vi "AppendNewPackets.vi"(6 "SampleLen":i32, 7 "SamplesInPacketNrLen":i32, 8 "ErrorIn":errorcluster, 9 "PacketsNum":u32, 10 "PacketsIn":T1[][](array[typedef]), 11 "FrameIn":string) -> (0 "ErrorOut":errorcluster, 2 "FrameOut":string, 3 "PacketsOut":T1[][](array[typedef]))   [LabVIEW 2016]
doc: "Convert input frame (string) and append new packets to the packet array. \n\nIf error occurs or is at the input, the VI ends execution."
uses:
  FallSensor/Sample.ctl
  FallSensor/Data.ctl
  FallSensor/DataType.ctl
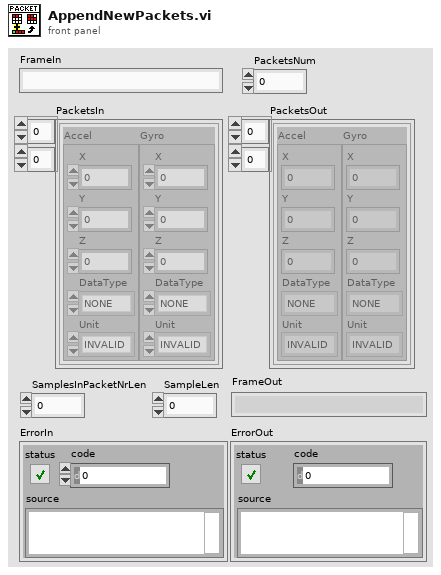
[diagram p1: front panel]
types:
  T1 = typedef "Sample.ctl" = cluster{"Accel":T2, "Gyro":T2}
  T2 = typedef "Data.ctl" = cluster{"X":dbl, "Y":dbl, "Z":dbl, "DataType":T3, "Unit":enum16{"INVALID", "g", "°/sec"}}
  T3 = typedef "DataType.ctl" = enum16{"NONE", "ACCEL", "GYRO"}
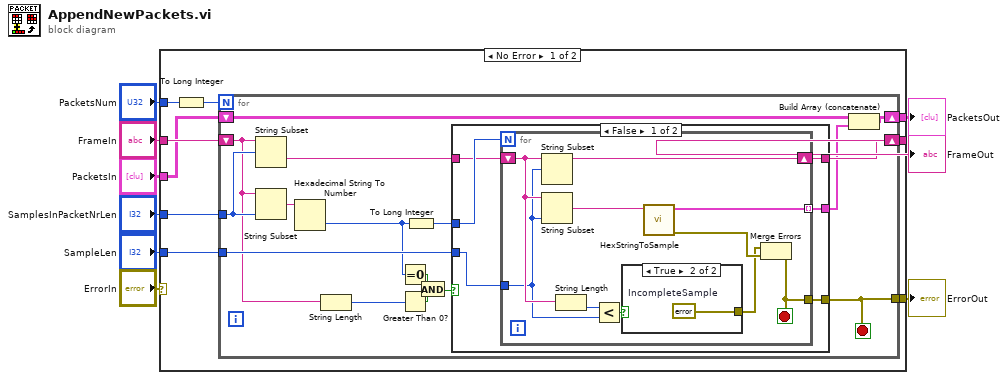
[diagram p0: block diagram]
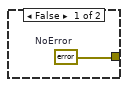
[diagram p2: hidden frame]
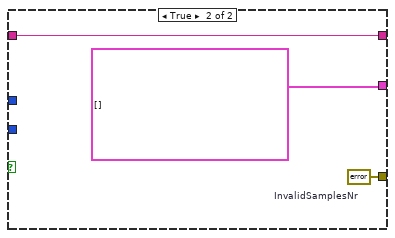
[diagram p3: hidden frame]
diagram:
  n1 = case shown="No Error" "ErrorIn" {
    selector: "ErrorIn" -> [_ w58]
    tunnel: [w18 w57] -> w9
    tunnel: "FrameIn" -> [w17 w56]
    tunnel: "PacketsIn" -> [w16 w57]
    tunnel: "PacketsNum" -> [w14 _]
    tunnel: [w10 w58] -> w4
    tunnel: "SamplesInPacketNrLen" -> [w13 _]
    tunnel: "SampleLen" -> [w12 _]
    tunnel: [w11 w56] -> w1
    frame No Error {
      n2 = To Long Integer(number=w14) -> (32bit integer=w15:i32)
      n3 = for {
        N: w15 -> [_]
        shift-right: [w34] -> w18
        shift-left: w16 -> [w33]
        tunnel: w13 -> [w31]
        tunnel: w12 -> [w30]
        shift-right: [w28] -> w11
        shift-left: w17 -> [w23]
        tunnel: [w25] -> w10
        stop <- w25 stop-if-true
        n4 = String Subset(string=w23, offset (0)=w31) -> (substring=w29:string)  [unwired: 1 in]
        n5 = String Subset(string=w23, length (rest)=w31) -> (substring=w32:string)  [unwired: 1 in]
        n6 = Hexadecimal String To Number ("HexStringToNumber")(string=w32) -> (number=w27:u32)  [unwired: 2 in, 1 out]
        n7 = String Length(string=w23) -> (length=w22:i32)
        n8 = Equal To 0?(x=w27) -> (x = 0?=w19:bool)
        n9 = Greater Than 0?(x=w22) -> (x > 0?=w20:bool)
        n10 = To Long Integer(number=w27) -> (32bit integer=w26:i32)
        n11 = And(x=w19, y=w20) -> (x .and. y?=w21:bool)
        n12 = case shown="False" w21 {
          tunnel: [w36 w55] -> w25
          tunnel: w30 -> [w38 _]
          tunnel: w29 -> [w39 w54]
          tunnel: [w37 w54] -> w28
          tunnel: w26 -> [w40 _]
          tunnel: [w35 T1[] []] -> w24
          frame False {
            n13 = for {
              N: w40 -> [_]
              tunnel: w38 -> [w45]
              shift-right: [w50] -> w37
              shift-left: w39 -> [w47]
              tunnel: [w43] -> w36
              tunnel: [w48] -> w35 mode=indexing
              stop <- w43 stop-if-true
              n14 = String Subset(string=w47, offset (0)=w45) -> (substring=w50:string)  [unwired: 1 in]
              n15 = String Subset(string=w47, length (rest)=w45) -> (substring=w49:string)  [unwired: 1 in]
              n16 = String Length(string=w47) -> (length=w46:i32)
              n17 = Less?(x=w46, y=w45) -> (x < y?=w44:bool)
              n18 = case shown="True" w44 {
                tunnel: [w51 w52] -> w41
                frame False {
                  w51 = errorcluster {"status"=FALSE, "code"=0, "source"=""}  # NoError
                }
                frame True {
                  w52 = errorcluster {"status"=TRUE, "code"=5, "source"="Incomplete sample"}  # IncompleteSample
                }
              }
              n19 = call "HexStringToSample.vi"("StringIn"=w49) -> ("ErrorOut"=w42:errorcluster, "Sample"=w48:T1)  [unwired: 8 in, 1 out]
              n20 = Merge Errors(w41, w42) -> (w43:errorcluster)
            }
          }
          frame True {
            w55 = errorcluster {"status"=TRUE, "code"=3, "source"="Invalid samples number"}  # InvalidSamplesNr
          }
        }
        n21 = Build Array (concatenate)(w33, w24) -> (w34:T1[][])
      }
    }
    frame Error {
    }
  }
  "PacketsOut" <- w9
  "ErrorOut" <- w4
  "FrameOut" <- w1
